vi "Read Driver Class.vi"(8 "error in":errorcluster, 11 "Plugin_Controller in":refnum<class "Plugin_Controller.lvclass">) -> (0 "error out":errorcluster, 2 "Plugin.lvlib:Plugin_Driver.lvclass":refnum<class "Plugin_Driver.lvclass">, 3 "Plugin_Controller out":refnum<class "Plugin_Controller.lvclass">)   [LabVIEW 2020, in "Plugin.lvlib" / "Plugin_Controller.lvclass"]
doc: "Read Driver class"
uses:
  Plugin_Controller.lvclass
  Plugin_Driver/Plugin_Driver.lvclass
  Plugin_Controller.lvclass/Plugin_Controller.ctl
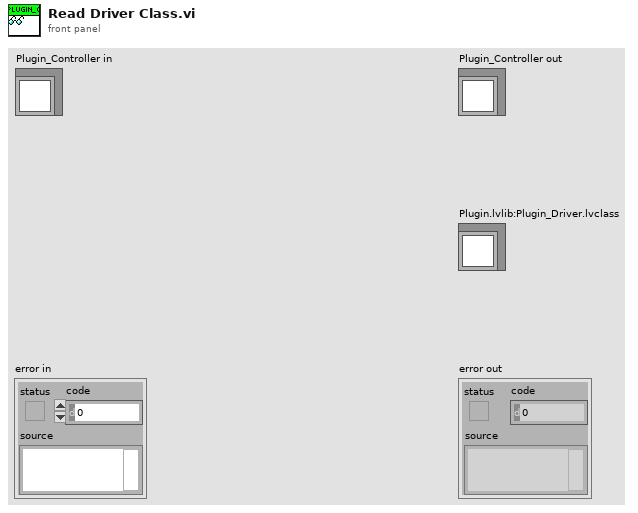
[diagram p1: front panel]
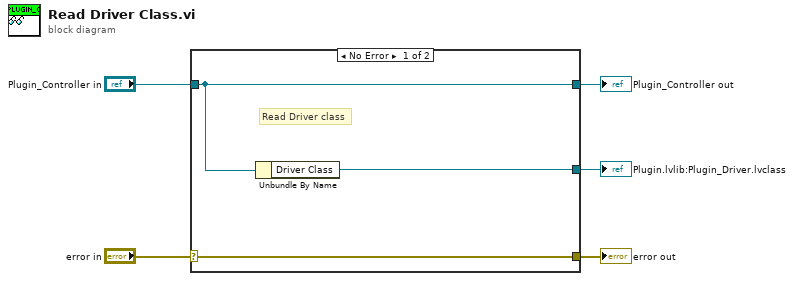
[diagram p0: block diagram]
diagram:
  n1 = case shown="No Error" "error in" {
    selector: "error in" -> [w8 w9]
    tunnel: [w8 w9] -> w4
    tunnel: [w7 w10] -> w2
    tunnel: "Plugin_Controller in" -> [w7 w10]
    tunnel: [w6 _] -> w1
    frame No Error {
      # "Read Driver class"
      n2 = Unbundle By Name(w7) -> ("Driver Class"=w6:refnum<class "Plugin_Driver.lvclass">)
    }
    frame Error {
    }
  }
  "error out" <- w4
  "Plugin_Controller out" <- w2
  "Plugin.lvlib:Plugin_Driver.lvclass" <- w1
